vi "TypeConv_Register Existing Identities.vi"(7 "Category":T1, 9 "Classes":T2[](array[typedef]), 10 "Existing Class Ref Map":variant) -> ()   [LabVIEW 2013]
uses:
  Data Structures/JSON/Class.ctl
  Data Structures/JSON/Enum.ctl
  Data Structures/JSON/Enum Value.ctl
  Data Structures/JSON/Method.ctl
  Data Structures/JSON/Param.ctl
  Data Structures/JSON/Property.ctl
  Category.ctl
  Action.ctl
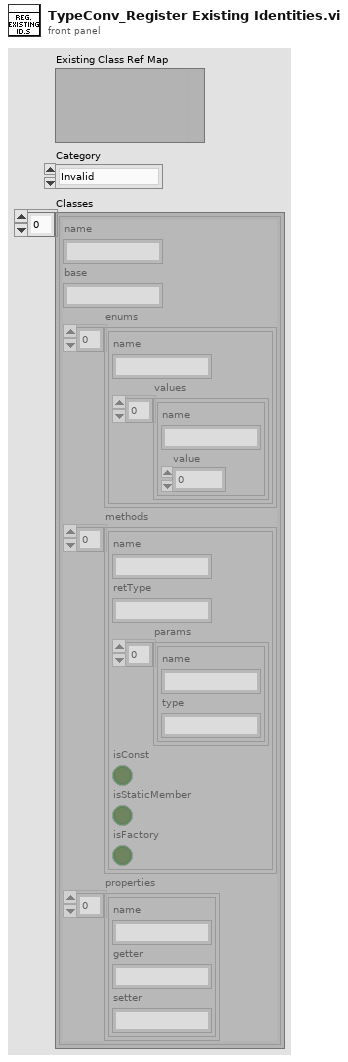
[diagram p1: front panel]
types:
  T1 = typedef "Category.ctl" = enum16{"Invalid", "Void", "Boolean", "Numeric", "Enum", "SimpleStruct", "OpaqueStruct", "SimpleIdentity", "QObject", "SimpleContainer", "FullArray"}
  T2 = typedef "Class.ctl" = cluster{"name":string, "base":string, "enums":T3[], "methods":T5[], "properties":T7[]}
  T3 = typedef "Enum.ctl" = cluster{"name":string, "values":T4[]}
  T4 = typedef "Enum Value.ctl" = cluster{"name":string, "value":i32}
  T5 = typedef "Method.ctl" = cluster{"name":string, "retType":string, "params":T6[], "isConst":bool, "isStaticMember":bool, "isFactory":bool}
  T6 = typedef "Param.ctl" = cluster{"name":string, "type":string}
  T7 = typedef "Property.ctl" = cluster{"name":string, "getter":string, "setter":string}
  T8 = typedef "Action.ctl" = enum16{"Register Type", "Register Projection", "Obtain Writer", "Get Projection"}
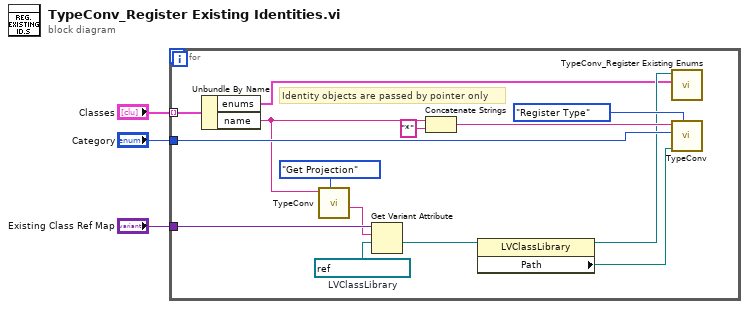
[diagram p0: block diagram]
diagram:
  n1 = for {
    tunnel: "Classes" -> [w14] mode=indexing
    tunnel: "Existing Class Ref Map" -> [w7]
    tunnel: "Category" -> [w13]
    w5 = refnum<vi> refnum  # LVClassLibrary
    # "Identity objects are passed by pointer only"
    n2 = Unbundle By Name(w14) -> ("enums"=w10:T3[], "name"=w8:string)
    n3 = call "TypeConv.vi"("Action"=Action."Get Projection", "Type Name"=w8) -> ("Projection Out"=w6:string)  [unwired: 7 in, 2 out]
    n4 = Get Variant Attribute(Variant=w7, name=w6, default value (empty Variant)=w5) -> (value=w4:refnum<vi>)  [unwired: 1 in, 3 out]
    n5 = Concatenate Strings(w8, "*" ("string")) -> (w16:string)
    n6 = property class="LVClassLibrary"(reference=w4) -> (reference out=w11:refnum<vi>, "Path"=w12:path)  [unwired: 1 in, 1 out]
    n7 = call "TypeConv_Register Existing Enums.vi"("Enums"=w10, "Owning Lib"=w11) -> ()  [unwired: 9 in, 1 out]
    n8 = call "TypeConv.vi"("Action"=Action."Register Type", "Type Path"=w12, "Category"=w13, "Type Name"=w16) -> ()  [unwired: 5 in, 3 out]
  }
